vi "CSC-Remote_DisplayCSC.vi"(4 "AnkleTraj":dbl[][](array[numeric]), 5 "ClosePt":dbl[](array[numeric]), 6 "Init?":bool, 7 "Field Force":dbl[](array[numeric]), 8 "error in (no error)":errorcluster, 9 "AxisSetting":T1={"AxisLabel"=["x ", "y", "z "], "AxisMax"=[0.6, 0.7, 0.2], "AxisMin"=[-0.4, -0.3, -0.8]}, 10 "3D graph in":refnum<k7>, 11 "CSC in":refnum<class "CableSerialChain.lvclass">) -> (0 "error out":errorcluster, 1 "LastPlotNum":i32=1, 2 "3D graph out":refnum<k7>, 3 "CSC out":refnum<class "CableSerialChain.lvclass">)   [LabVIEW 2015, in "CSC-Remote.lvclass"]
uses:
  CSC-Remote.lvclass
  CableSerialChain/CableSerialChain.lvclass
  <vilib>/Platform/NI_3dgraph.lvlib
  <vilib>/ptbypt/NI_PtbyPt.lvlib
panel:
  out "EndEffInGCS":dbl[](array[numeric]) format="%#.6f"
  in  "sample length":i32=15
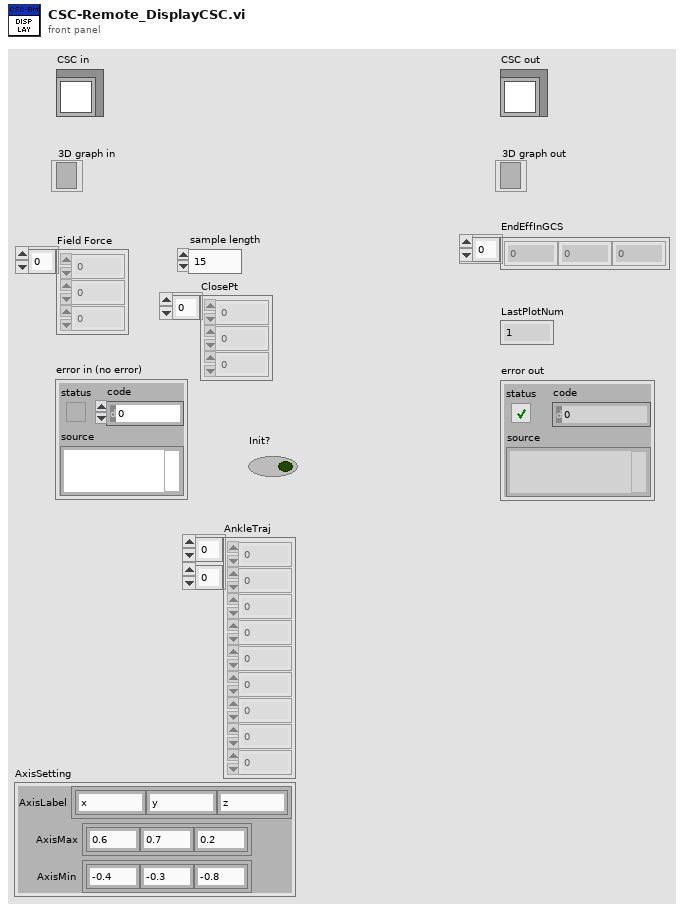
[diagram p1: front panel]
types:
  T1 = cluster{"AxisLabel":string[], "AxisMax":dbl[], "AxisMin":dbl[]}
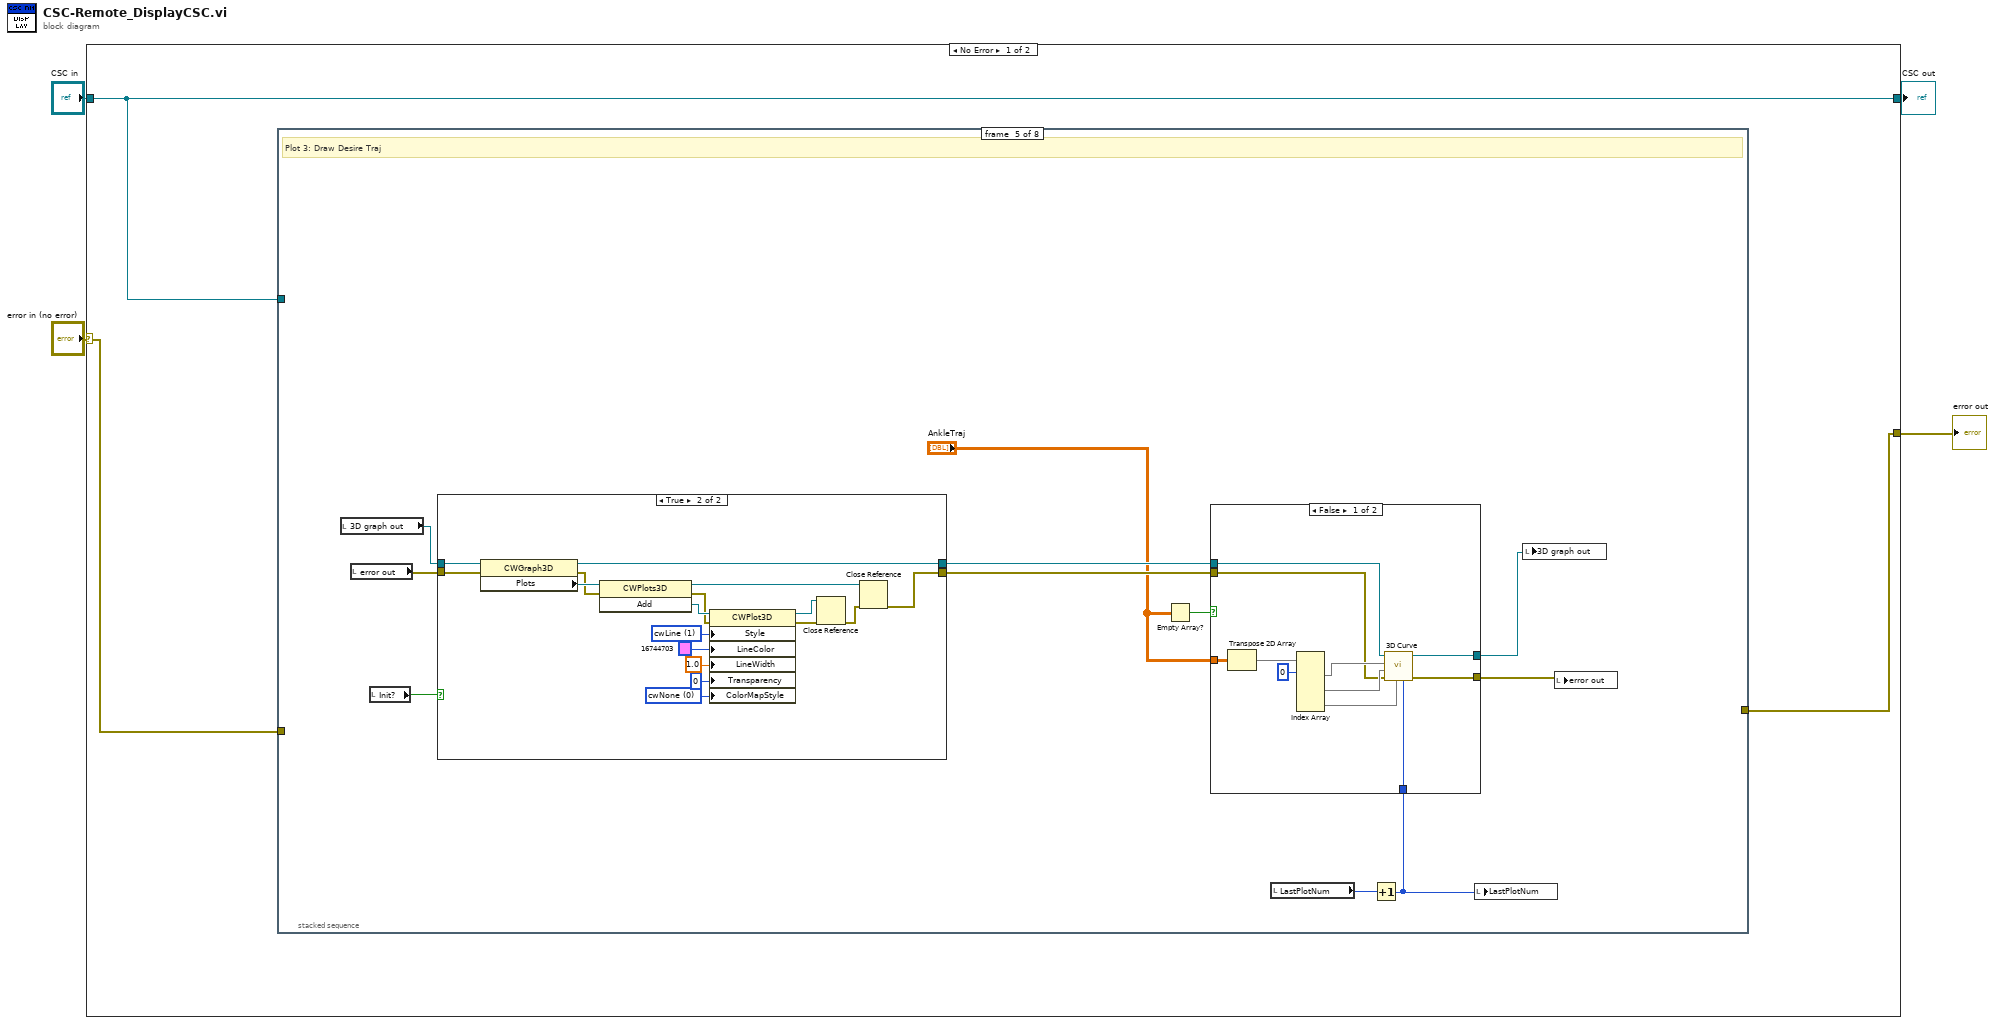
[diagram p0: block diagram]
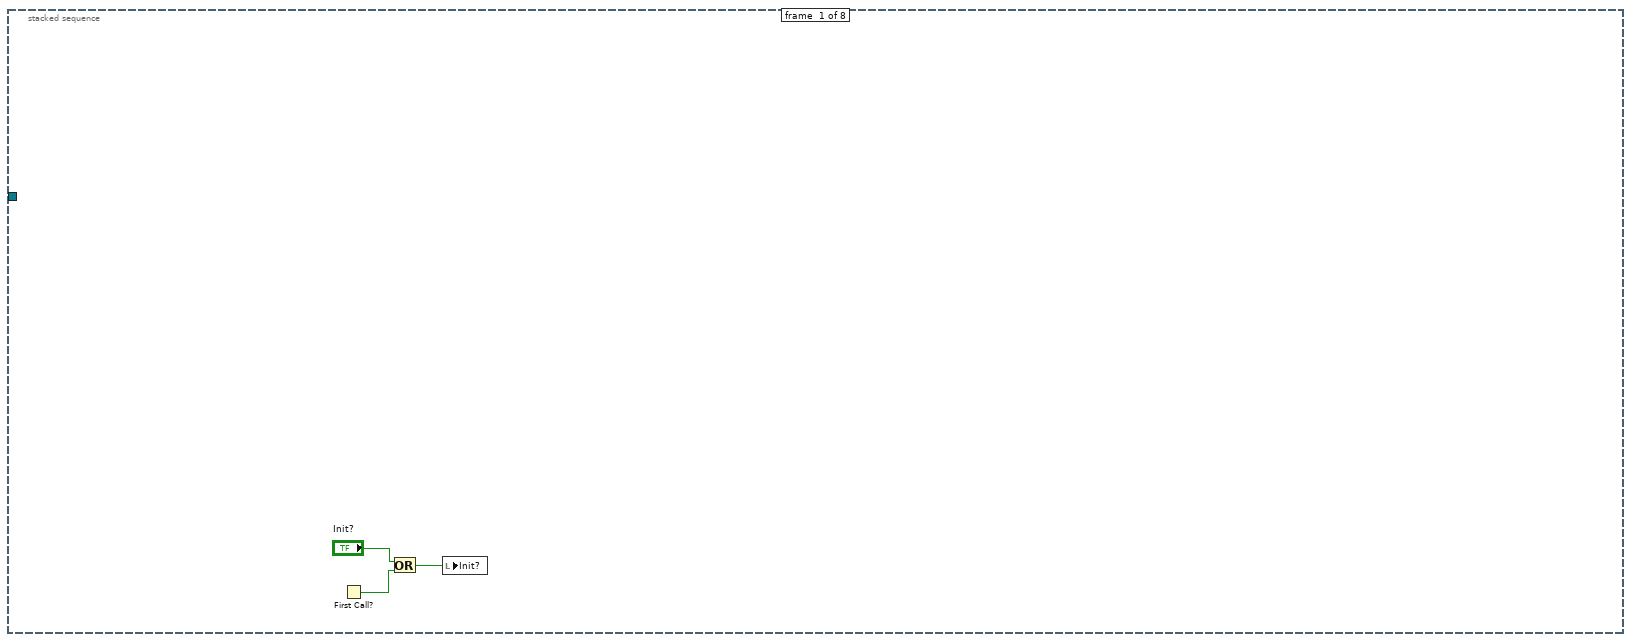
[diagram p2: hidden frame]
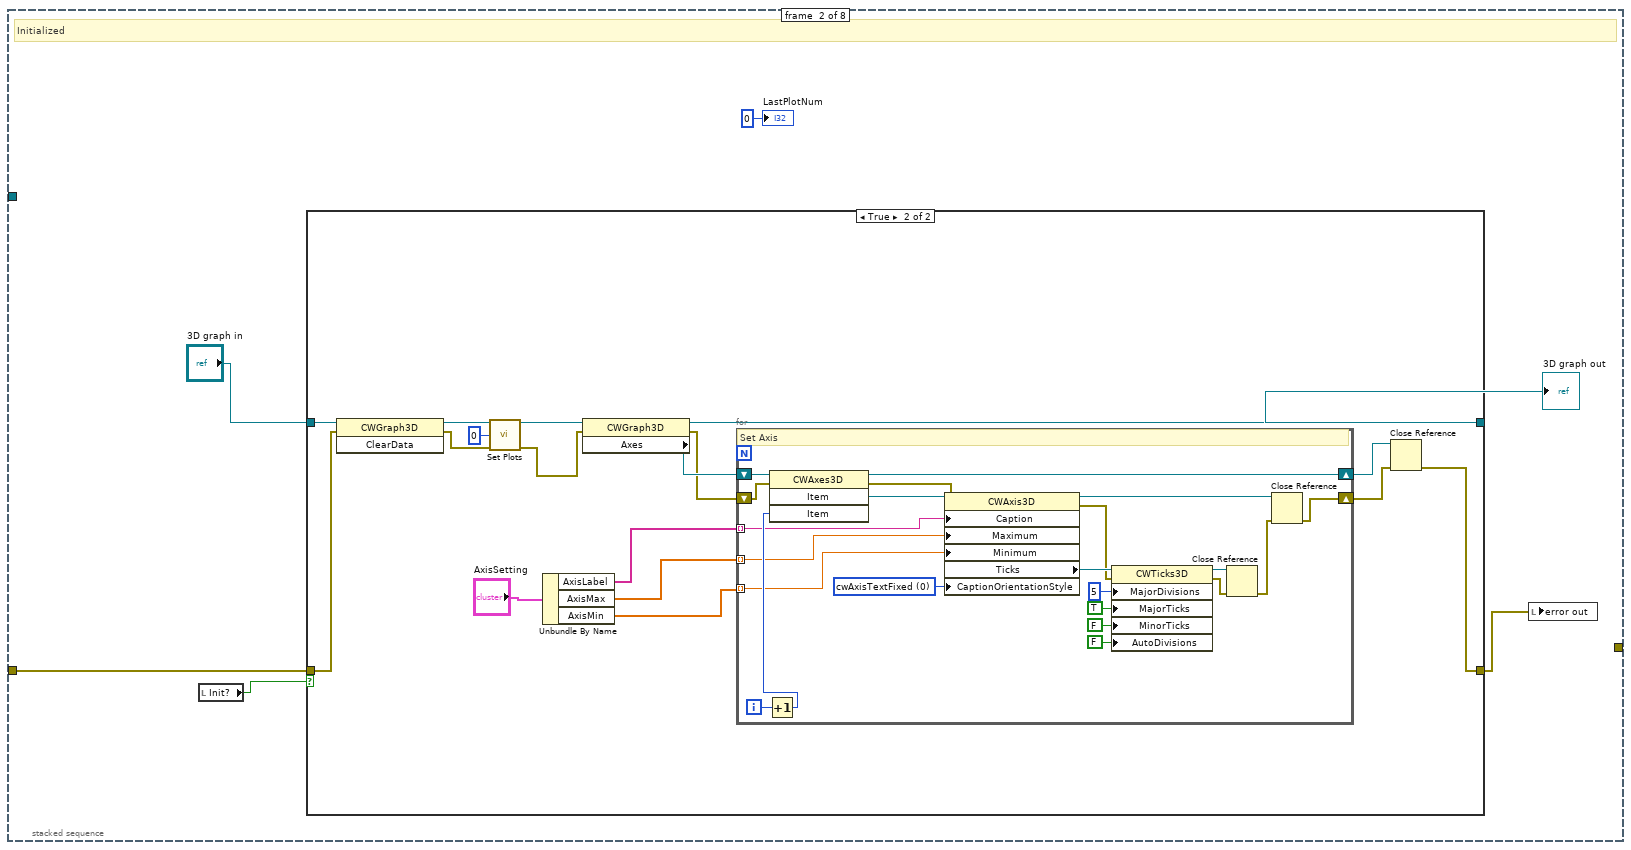
[diagram p3: hidden frame]
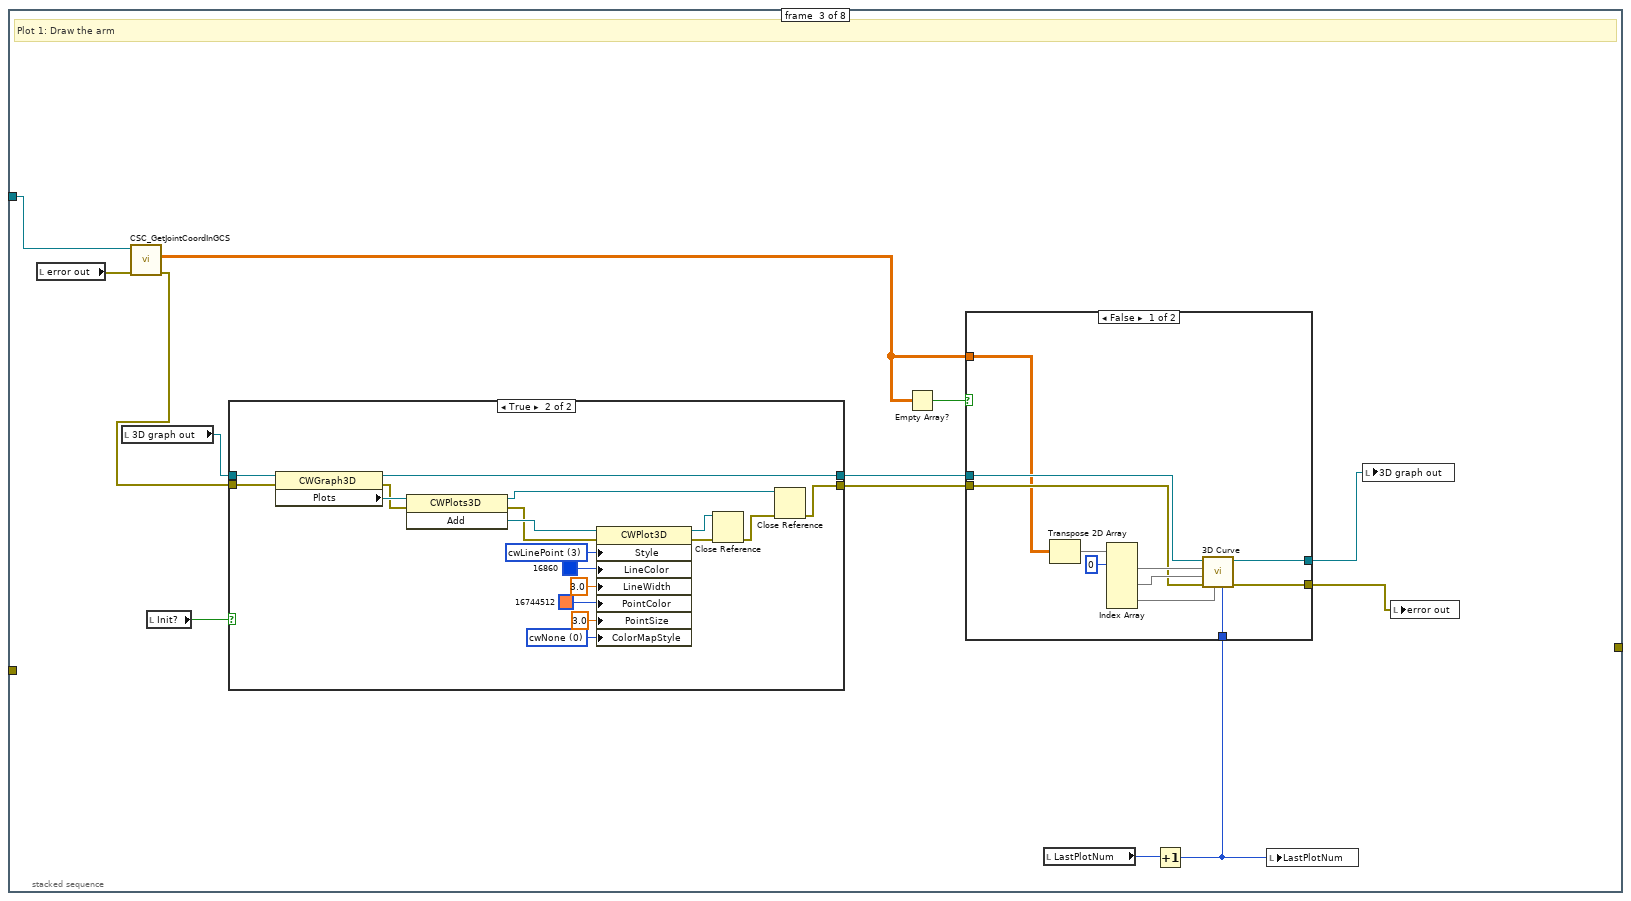
[diagram p5: hidden frame]
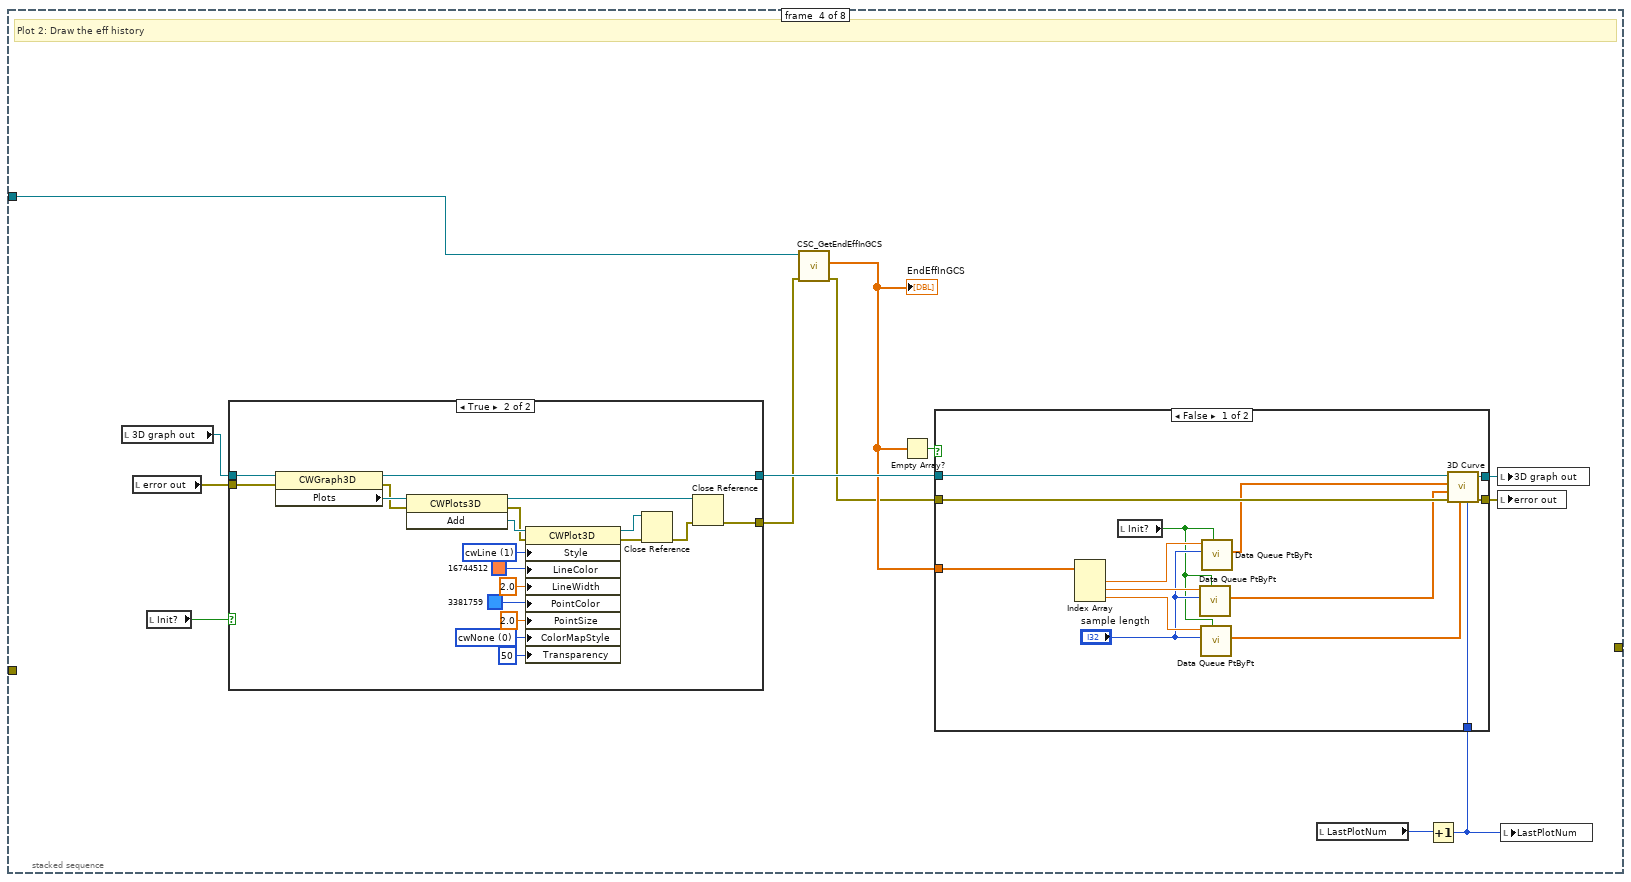
[diagram p8: hidden frame]
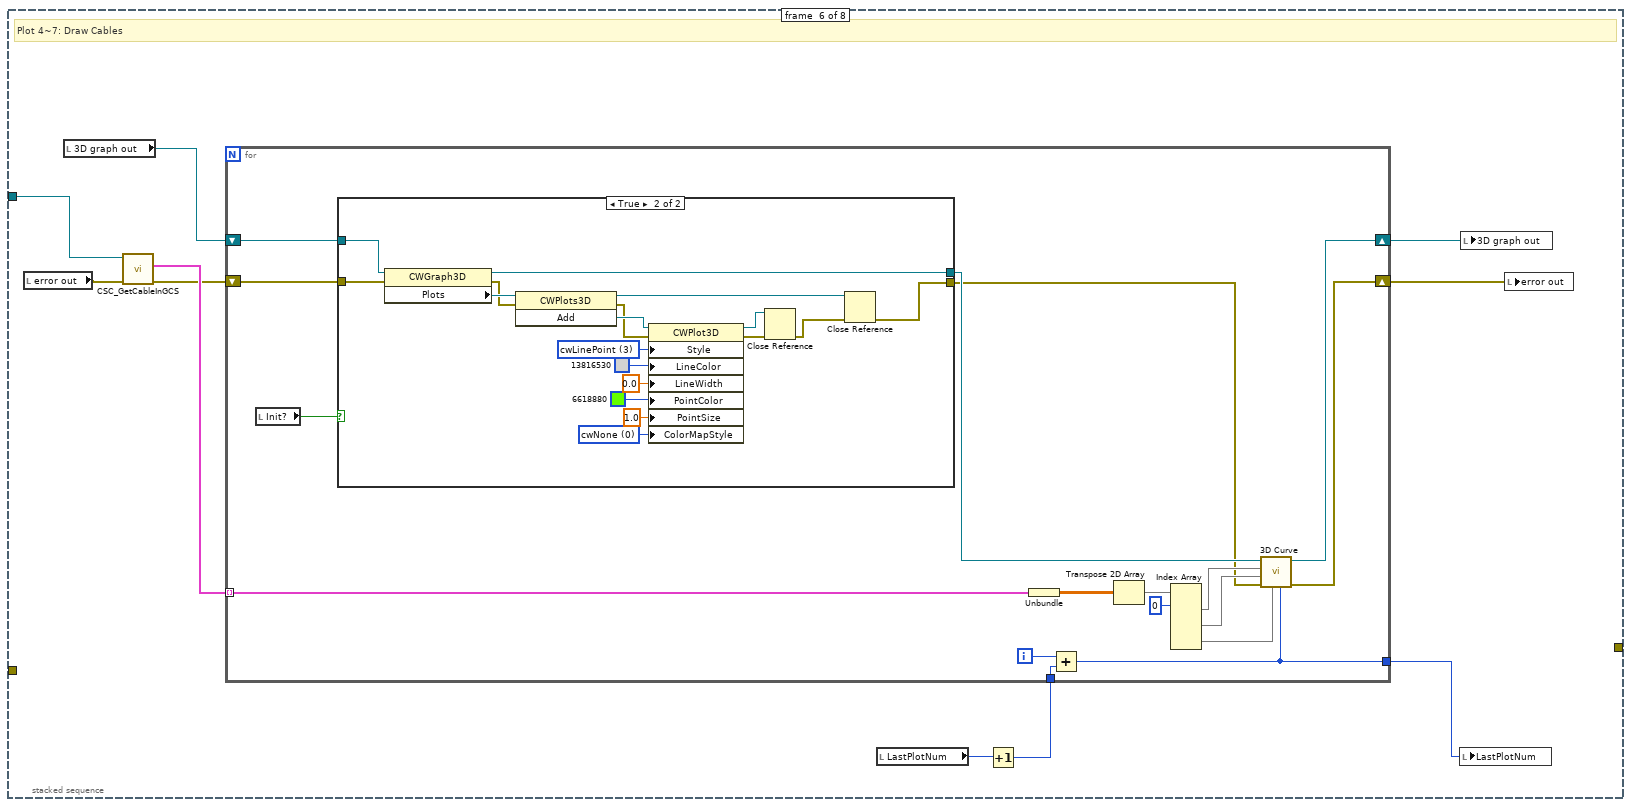
[diagram p13: hidden frame]
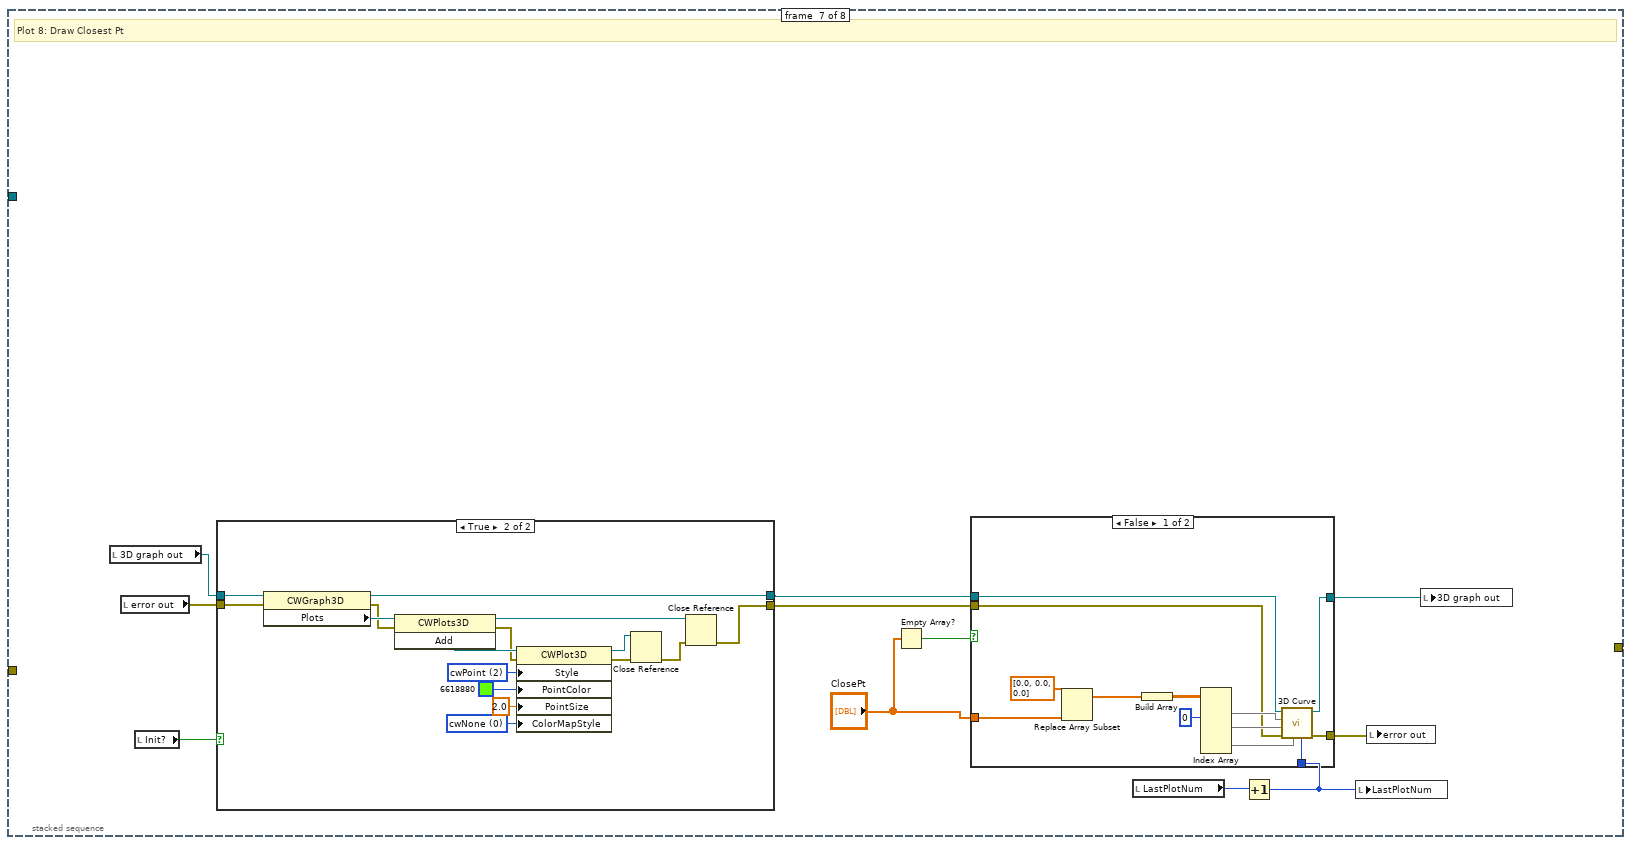
[diagram p15: hidden frame]
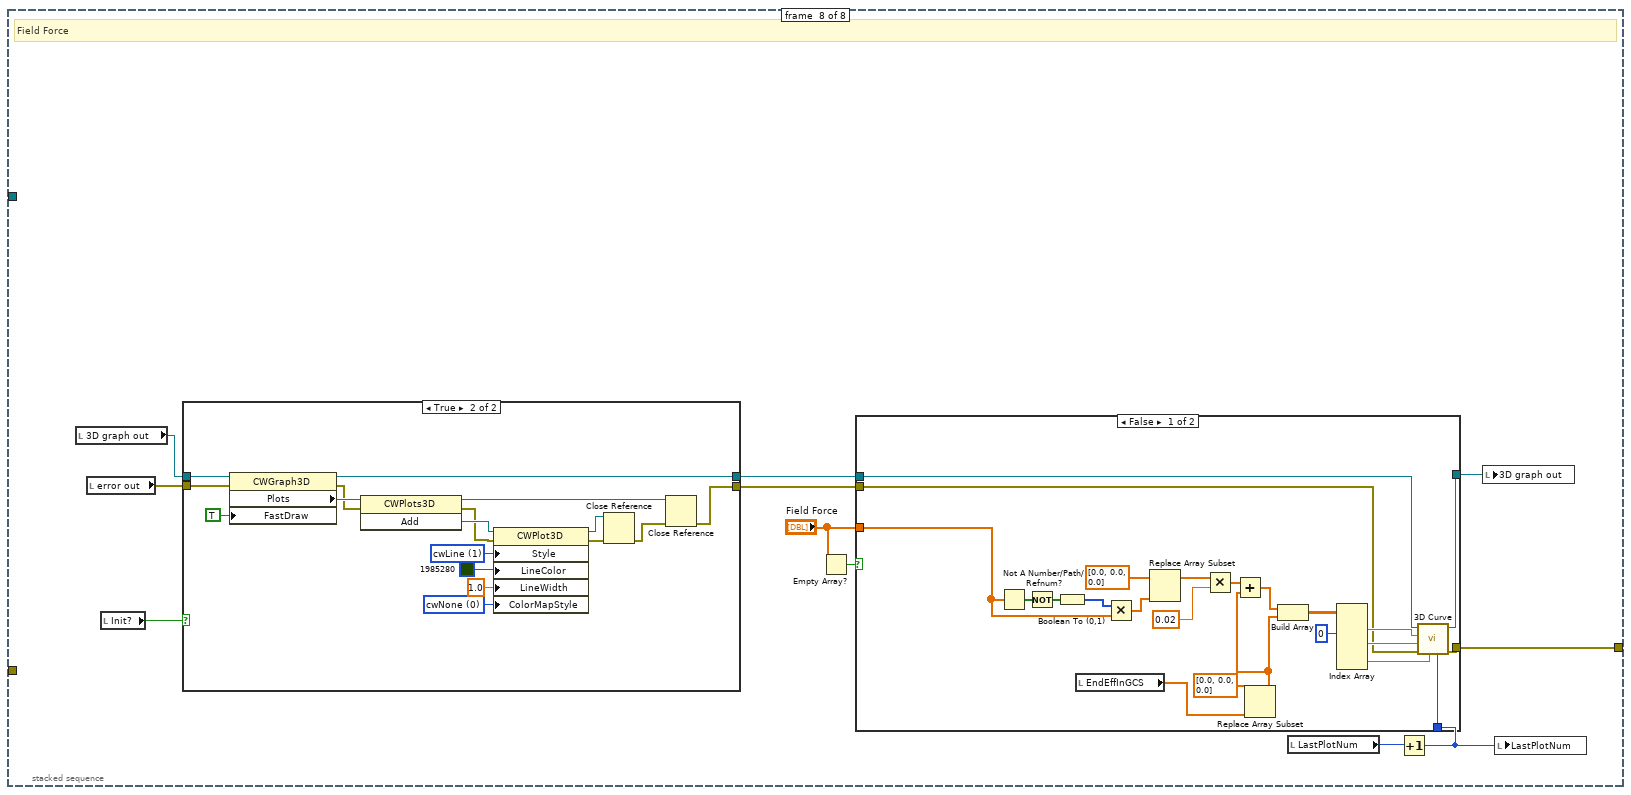
[diagram p18: hidden frame]
diagram:
  n1 = case shown="No Error" "error in (no error)" {
    selector: "error in (no error)" -> [w6 w344]
    tunnel: [w7 w344] -> w1
    tunnel: [w5 w343] -> w2
    tunnel: "CSC in" -> [w5 w343]
    frame No Error {
      n2 = stacked-sequence {
        tunnel: [_ _ _ _ _ _ _ w288] -> w7
        tunnel: w6 -> [_ w12 _ _ _ _ _ _]
        tunnel: w5 -> [_ _ w68 w116 _ w203 _ _]
        frame #0 {
          n3 = First Call?() -> (First Call?: T/F=w10:bool)
          n4 = Or(x="Init?", y=w10) -> (x .or. y?=w8:bool)
          n5 = local write "Init?"(w8) -> ()
        }
        frame #1 {
          # "Initialized"
          n6 = local read "Init?"() -> (w11:bool)
          n7 = case shown="True" w11 {
            tunnel: "3D graph in" -> [w18 w32]
            tunnel: [w18 w28] -> w15
            tunnel: [w17 w23] -> w13
            tunnel: w12 -> [w17 w30]
            frame False {
            }
            frame True {
              n8 = invoke class="CWGraph3D" method="ClearData"(reference=w32, error in=w30) -> (reference out=w31:refnum<k7>, error out=w29:errorcluster)  [unwired: 1 in, 1 out]
              n9 = call <vilib>:"Set Plots.vi"("3D graph"=w31, "# of plots(1)"=0, "error in (no error)"=w29) -> ("3D graph out"=w33:refnum<k7>, "error out"=w24:errorcluster)  [unwired: 11 in]
              n10 = Unbundle By Name("AxisSetting") -> ("AxisLabel"=w21:string[], "AxisMax"=w20:dbl[], "AxisMin"=w19:dbl[])
              n11 = property class="CWGraph3D"(reference=w33, error in=w24) -> (reference out=w28:refnum<k7>, error out=w25:errorcluster, "Axes"=w34:refnum<k7>)
              n12 = for {
                shift-right: [w44] -> w26
                shift-left: w34 -> [w57]
                shift-right: [w45] -> w27
                shift-left: w25 -> [w42]
                tunnel: w21 -> [w38] mode=indexing
                tunnel: w20 -> [w37] mode=indexing
                tunnel: w19 -> [w36] mode=indexing
                i -> [w40]
                w41 = 0 items=["cwAxisTextFixed", "cwAxisTextFaceCamera"] ("CaptionOrientationStyle")
                # "Set Axis"
                n13 = Increment(x=w40) -> (x+1=w39:i32)
                n14 = invoke class="CWAxes3D" method="Item"(reference=w57, error in=w42, "Item"=w39) -> (reference out=w44:refnum<k7>, error out=w43:errorcluster, "Item"=w56:refnum<k7>)  [unwired: 1 in, 1 out]
                n15 = property class="CWAxis3D"(reference=w56, error in=w43, "Caption"=w38, "Maximum"=w37, "Minimum"=w36, "CaptionOrientationStyle"=w41) -> (reference out=w46:refnum<k7>, error out=w49:errorcluster, "Ticks"=w55:refnum<k7>)
                n16 = property class="CWTicks3D"(reference=w55, error in=w49, "MajorDivisions"=5, "MajorTicks"=TRUE, "MinorTicks"=FALSE, "AutoDivisions"=FALSE) -> (reference out=w48:refnum<k7>, error out=w50:errorcluster)
                n17 = Close Reference(reference=w48, error in (no error)=w50) -> (error out=w47:errorcluster)
                n18 = Close Reference(reference=w46, error in (no error)=w47) -> (error out=w45:errorcluster)
              }
              n19 = Close Reference(reference=w26, error in (no error)=w27) -> (error out=w23:errorcluster)
            }
          }
          "3D graph out" <- w15
          n20 = local write "error out"(w13) -> ()
          "LastPlotNum" <- 0 ("LastPlotNum 2")
        }
        frame #2 {
          # "Plot 1: Draw the arm"
          n21 = local read "error out"() -> (w60:errorcluster)
          n22 = local read "3D graph out"() -> (w66:refnum<k7>)
          n23 = call "CSC_GetJointCoordInGCS.vi"("error in (no error)"=w60, "C-Alex in"=w68) -> ("error out"=w59:errorcluster, "Joint Coord in GCS"=w58:dbl[][])  [unwired: 6 in, 2 out]
          n24 = local read "Init?"() -> (w62:bool)
          n25 = case shown="True" w62 {
            tunnel: w59 -> [w84 w97]
            tunnel: w66 -> [w85 w92]
            tunnel: [w85 w91] -> w65
            tunnel: [w84 w86] -> w64
            frame False {
            }
            frame True {
              w90 = 0 items=["cwNone", "cwShaded", "cwColorSpectrum", "cwGrayScale", "cwCustom"] ("ColorMapStyle")
              w103 = 3 items=["cwLine"=1, "cwPoint"=2, "cwLinePoint"=3, "cwHiddenLine"=4, "cwSurface"=5, "cwSurfaceLine"=6, "cwSurfaceNormal"=7, "cwContourLine"=8, "cwSurfaceContour"=9] ("Style")
              n26 = property class="CWGraph3D"(reference=w92, error in=w97) -> (reference out=w91:refnum<k7>, error out=w100:errorcluster, "Plots"=w101:refnum<k7>)
              n27 = invoke class="CWPlots3D" method="Add"(reference=w101, error in=w100) -> (reference out=w88:refnum<k7>, error out=w89:errorcluster, "Add"=w102:refnum<k7>)  [unwired: 1 in]
              n28 = property class="CWPlot3D"(reference=w102, error in=w89, "Style"=w103, "LineColor"=u32 16860, "LineWidth"=3.0, "PointColor"=u32 16744512, "PointSize"=3.0 ("LineWidth"), "ColorMapStyle"=w90) -> (reference out=w98:refnum<k7>, error out=w99:errorcluster)
              n29 = Close Reference(reference=w98, error in (no error)=w99) -> (error out=w87:errorcluster)
              n30 = Close Reference(reference=w88, error in (no error)=w87) -> (error out=w86:errorcluster)
            }
          }
          n31 = Empty Array?(array=w58) -> (empty?=w61:bool)
          n32 = local read "LastPlotNum"() -> (w70:i32)
          n33 = Increment(x=w70) -> (x+1=w69:i32)
          n34 = case shown="False" w61 {
            tunnel: [w76 w83] -> w67
            tunnel: w65 -> [w75 w83]
            tunnel: w64 -> [w74 w82]
            tunnel: [w73 w82] -> w63
            tunnel: w69 -> [w72 _]
            tunnel: w58 -> [w71 _]
            frame False {
              n35 = Transpose 2D Array(2D array=w71) -> (transposed array=w77:dbl[][])
              n36 = Index Array(array=w77, index (row) #1=0 ("index (row)")) -> (element #1=w79:dbl[], element #2=w80:dbl[], element #3=w81:dbl[])  [unwired: 5 in]
              n37 = call <vilib>:"3D Curve.vi"("plot number (1)"=w72, "z vector"=w81, "error in (no error)"=w74, "y vector"=w80, "x vector"=w79, "3D graph"=w75) -> ("error out"=w73:errorcluster, "3D graph out"=w76:refnum<k7>)  [unwired: 4 in]
            }
            frame True {
            }
          }
          n38 = local write "LastPlotNum"(w69) -> ()
          n39 = local write "3D graph out"(w67) -> ()
          n40 = local write "error out"(w63) -> ()
        }
        frame #3 {
          # "Plot 2: Draw the eff history"
          n41 = local read "3D graph out"() -> (w111:refnum<k7>)
          n42 = local read "error out"() -> (w112:errorcluster)
          n43 = local read "Init?"() -> (w108:bool)
          n44 = case shown="True" w108 {
            tunnel: w112 -> [w133 w146]
            tunnel: w111 -> [w134 w141]
            tunnel: [w134 w140] -> w110
            tunnel: [w133 w135] -> w105
            frame False {
            }
            frame True {
              w139 = 0 items=["cwNone", "cwShaded", "cwColorSpectrum", "cwGrayScale", "cwCustom"] ("ColorMapStyle")
              w153 = 1 items=["cwLine"=1, "cwPoint"=2, "cwLinePoint"=3, "cwHiddenLine"=4, "cwSurface"=5, "cwSurfaceLine"=6, "cwSurfaceNormal"=7, "cwContourLine"=8, "cwSurfaceContour"=9] ("Style")
              n45 = property class="CWGraph3D"(reference=w141, error in=w146) -> (reference out=w140:refnum<k7>, error out=w150:errorcluster, "Plots"=w151:refnum<k7>)
              n46 = invoke class="CWPlots3D" method="Add"(reference=w151, error in=w150) -> (reference out=w149:refnum<k7>, error out=w137:errorcluster, "Add"=w152:refnum<k7>)  [unwired: 1 in]
              n47 = property class="CWPlot3D"(reference=w152, error in=w137, "Style"=w153, "LineColor"=u32 16744512, "LineWidth"=2.0, "PointColor"=u32 3381759, "PointSize"=2.0 ("LineWidth"), "ColorMapStyle"=w139, "Transparency"=50) -> (reference out=w147:refnum<k7>, error out=w148:errorcluster)
              n48 = Close Reference(reference=w147, error in (no error)=w148) -> (error out=w136:errorcluster)
              n49 = Close Reference(reference=w149, error in (no error)=w136) -> (error out=w135:errorcluster)
            }
          }
          n50 = call "CSC_GetEndEffInGCS.vi"("error in (no error)"=w105, "CSC in"=w116) -> ("error out"=w104:errorcluster, "EndEffInGCS"=w106:dbl[])  [unwired: 5 in, 3 out]
          "EndEffInGCS" <- w106
          n51 = Empty Array?(array=w106) -> (empty?=w107:bool)
          n52 = local read "LastPlotNum"() -> (w114:i32)
          n53 = Increment(x=w114) -> (x+1=w115:i32)
          n54 = case shown="False" w107 {
            tunnel: [w130 w132] -> w113
            tunnel: w110 -> [w129 w132]
            tunnel: w104 -> [w128 w131]
            tunnel: [w127 w131] -> w109
            tunnel: w115 -> [w126 _]
            tunnel: w106 -> [w117 _]
            frame False {
              n55 = Index Array(array=w117) -> (element #1=w123:dbl, element #2=w124:dbl, element #3=w125:dbl)  [unwired: 3 in]
              n56 = local read "Init?"() -> (w118:bool)
              n57 = call <vilib>:"Data Queue PtByPt.vi"("initialize"=w118, "sample length"="sample length", "input data point"=w124) -> ("Current Queue"=w120:dbl[])  [unwired: 4 in, 4 out]
              n58 = call <vilib>:"Data Queue PtByPt.vi"("initialize"=w118, "sample length"="sample length", "input data point"=w125) -> ("Current Queue"=w119:dbl[])  [unwired: 4 in, 4 out]
              n59 = call <vilib>:"Data Queue PtByPt.vi"("initialize"=w118, "sample length"="sample length", "input data point"=w123) -> ("Current Queue"=w121:dbl[])  [unwired: 4 in, 4 out]
              n60 = call <vilib>:"3D Curve.vi"("plot number (1)"=w126, "z vector"=w119, "error in (no error)"=w128, "y vector"=w120, "x vector"=w121, "3D graph"=w129) -> ("error out"=w127:errorcluster, "3D graph out"=w130:refnum<k7>)  [unwired: 4 in]
            }
            frame True {
            }
          }
          n61 = local write "3D graph out"(w113) -> ()
          n62 = local write "error out"(w109) -> ()
          n63 = local write "LastPlotNum"(w115) -> ()
        }
        frame #4 {
          # "Plot 3: Draw Desire Traj"
          n64 = local read "3D graph out"() -> (w160:refnum<k7>)
          n65 = local read "error out"() -> (w161:errorcluster)
          n66 = local read "Init?"() -> (w158:bool)
          n67 = case shown="True" w158 {
            tunnel: w161 -> [w178 w189]
            tunnel: w160 -> [w179 w186]
            tunnel: [w179 w185] -> w159
            tunnel: [w178 w180] -> w157
            frame False {
            }
            frame True {
              w183 = 0 items=["cwNone", "cwShaded", "cwColorSpectrum", "cwGrayScale", "cwCustom"] ("ColorMapStyle")
              w196 = 1 items=["cwLine"=1, "cwPoint"=2, "cwLinePoint"=3, "cwHiddenLine"=4, "cwSurface"=5, "cwSurfaceLine"=6, "cwSurfaceNormal"=7, "cwContourLine"=8, "cwSurfaceContour"=9] ("Style")
              n68 = property class="CWGraph3D"(reference=w186, error in=w189) -> (reference out=w185:refnum<k7>, error out=w193:errorcluster, "Plots"=w194:refnum<k7>)
              n69 = invoke class="CWPlots3D" method="Add"(reference=w194, error in=w193) -> (reference out=w192:refnum<k7>, error out=w182:errorcluster, "Add"=w195:refnum<k7>)  [unwired: 1 in]
              n70 = property class="CWPlot3D"(reference=w195, error in=w182, "Style"=w196, "LineColor"=u32 16744703, "LineWidth"=1.0, "Transparency"=0, "ColorMapStyle"=w183) -> (reference out=w190:refnum<k7>, error out=w191:errorcluster)
              n71 = Close Reference(reference=w190, error in (no error)=w191) -> (error out=w181:errorcluster)
              n72 = Close Reference(reference=w192, error in (no error)=w181) -> (error out=w180:errorcluster)
            }
          }
          n73 = Empty Array?(array="AnkleTraj") -> (empty?=w155:bool)
          n74 = local read "LastPlotNum"() -> (w164:i32)
          n75 = Increment(x=w164) -> (x+1=w163:i32)
          n76 = case shown="False" w155 {
            tunnel: "AnkleTraj" -> [w175 _]
            tunnel: [w169 w177] -> w162
            tunnel: w159 -> [w168 w177]
            tunnel: w163 -> [w167 _]
            tunnel: w157 -> [w166 w176]
            tunnel: [w165 w176] -> w156
            frame False {
              n77 = Transpose 2D Array(2D array=w175) -> (transposed array=w170:dbl[][])
              n78 = Index Array(array=w170, index (row) #1=0 ("index (row)")) -> (element #1=w172:dbl[], element #2=w173:dbl[], element #3=w174:dbl[])  [unwired: 5 in]
              n79 = call <vilib>:"3D Curve.vi"("plot number (1)"=w167, "z vector"=w174, "error in (no error)"=w166, "y vector"=w173, "x vector"=w172, "3D graph"=w168) -> ("error out"=w165:errorcluster, "3D graph out"=w169:refnum<k7>)  [unwired: 4 in]
            }
            frame True {
            }
          }
          n80 = local write "LastPlotNum"(w163) -> ()
          n81 = local write "3D graph out"(w162) -> ()
          n82 = local write "error out"(w156) -> ()
        }
        frame #5 {
          # "Plot 4~7: Draw Cables"
          n83 = local read "error out"() -> (w197:errorcluster)
          n84 = local read "3D graph out"() -> (w201:refnum<k7>)
          n85 = call "CSC_GetCableInGCS.vi"("error in (no error)"=w197, "C-Alex in"=w203) -> ("error out"=w198:errorcluster, "Cables Points"=w200:cluster{"PointInGCS":dbl[][]}[])  [unwired: 7 in, 1 out]
          n86 = local read "LastPlotNum"() -> (w206:i32)
          n87 = Increment(x=w206) -> (x+1=w205:i32)
          n88 = for {
            tunnel: w200 -> [w221] mode=indexing
            shift-right: [w219] -> w202
            shift-left: w201 -> [w213]
            tunnel: w205 -> [w211]
            tunnel: [w210] -> w204
            shift-right: [w208] -> w199
            shift-left: w198 -> [w207]
            i -> [w215]
            n89 = local read "Init?"() -> (w214:bool)
            n90 = case shown="True" w214 {
              tunnel: w207 -> [w225 w236]
              tunnel: [w224 w231] -> w212
              tunnel: [w225 w226] -> w209
              tunnel: w213 -> [w224 w229]
              frame False {
              }
              frame True {
                w230 = 0 items=["cwNone", "cwShaded", "cwColorSpectrum", "cwGrayScale", "cwCustom"] ("ColorMapStyle")
                w243 = 3 items=["cwLine"=1, "cwPoint"=2, "cwLinePoint"=3, "cwHiddenLine"=4, "cwSurface"=5, "cwSurfaceLine"=6, "cwSurfaceNormal"=7, "cwContourLine"=8, "cwSurfaceContour"=9] ("Style")
                n91 = property class="CWGraph3D"(reference=w229, error in=w236) -> (reference out=w231:refnum<k7>, error out=w240:errorcluster, "Plots"=w241:refnum<k7>)
                n92 = invoke class="CWPlots3D" method="Add"(reference=w241, error in=w240) -> (reference out=w239:refnum<k7>, error out=w228:errorcluster, "Add"=w242:refnum<k7>)  [unwired: 1 in]
                n93 = property class="CWPlot3D"(reference=w242, error in=w228, "Style"=w243, "LineColor"=u32 13816530, "LineWidth"=0.0, "PointColor"=u32 6618880, "PointSize"=1.0 ("LineWidth"), "ColorMapStyle"=w230) -> (reference out=w237:refnum<k7>, error out=w238:errorcluster)
                n94 = Close Reference(reference=w237, error in (no error)=w238) -> (error out=w227:errorcluster)
                n95 = Close Reference(reference=w239, error in (no error)=w227) -> (error out=w226:errorcluster)
              }
            }
            n96 = Unbundle(w221) -> ("PointInGCS"=w220:dbl[][])
            n97 = Add(x=w215, y=w211) -> (x+y=w210:i32)
            n98 = Transpose 2D Array(2D array=w220) -> (transposed array=w222:dbl[][])
            n99 = Index Array(array=w222, index (row) #1=0 ("index (row)")) -> (element #1=w218:dbl[], element #2=w217:dbl[], element #3=w216:dbl[])  [unwired: 5 in]
            n100 = call <vilib>:"3D Curve.vi"("plot number (1)"=w210, "z vector"=w216, "error in (no error)"=w209, "y vector"=w217, "x vector"=w218, "3D graph"=w212) -> ("error out"=w208:errorcluster, "3D graph out"=w219:refnum<k7>)  [unwired: 4 in]
          }
          n101 = local write "LastPlotNum"(w204) -> ()
          n102 = local write "3D graph out"(w202) -> ()
          n103 = local write "error out"(w199) -> ()
        }
        frame #6 {
          # "Plot 8: Draw Closest Pt"
          n104 = local read "3D graph out"() -> (w252:refnum<k7>)
          n105 = local read "error out"() -> (w253:errorcluster)
          n106 = local read "Init?"() -> (w251:bool)
          n107 = case shown="True" w251 {
            tunnel: w253 -> [w270 w280]
            tunnel: w252 -> [w271 w277]
            tunnel: [w271 w276] -> w250
            tunnel: [w270 w272] -> w247
            frame False {
            }
            frame True {
              w275 = 0 items=["cwNone", "cwShaded", "cwColorSpectrum", "cwGrayScale", "cwCustom"] ("ColorMapStyle")
              w287 = 2 items=["cwLine"=1, "cwPoint"=2, "cwLinePoint"=3, "cwHiddenLine"=4, "cwSurface"=5, "cwSurfaceLine"=6, "cwSurfaceNormal"=7, "cwContourLine"=8, "cwSurfaceContour"=9] ("Style")
              n108 = property class="CWGraph3D"(reference=w277, error in=w280) -> (reference out=w276:refnum<k7>, error out=w284:errorcluster, "Plots"=w285:refnum<k7>)
              n109 = invoke class="CWPlots3D" method="Add"(reference=w285, error in=w284) -> (reference out=w283:refnum<k7>, error out=w274:errorcluster, "Add"=w286:refnum<k7>)  [unwired: 1 in]
              n110 = property class="CWPlot3D"(reference=w286, error in=w274, "Style"=w287, "PointColor"=u32 6618880, "PointSize"=2.0 ("LineWidth"), "ColorMapStyle"=w275) -> (reference out=w281:refnum<k7>, error out=w282:errorcluster)
              n111 = Close Reference(reference=w281, error in (no error)=w282) -> (error out=w273:errorcluster)
              n112 = Close Reference(reference=w283, error in (no error)=w273) -> (error out=w272:errorcluster)
            }
          }
          n113 = Empty Array?(array="ClosePt") -> (empty?=w244:bool)
          n114 = local read "LastPlotNum"() -> (w249:i32)
          n115 = Increment(x=w249) -> (x+1=w248:i32)
          n116 = case shown="False" w244 {
            tunnel: "ClosePt" -> [w266 _]
            tunnel: [w259 w269] -> w254
            tunnel: w250 -> [w258 w269]
            tunnel: w248 -> [w257 _]
            tunnel: w247 -> [w256 w268]
            tunnel: [w255 w268] -> w246
            frame False {
              n117 = Replace Array Subset(array=dbl[] [0.0, 0.0, 0.0], new element=w266) -> (w265:dbl[])  [unwired: 1 in]
              n118 = Build Array(w265) -> (w264:dbl[][])
              n119 = Index Array(array=w264, index (col) #1=0 ("disabled index (col)")) -> (element #1=w262:dbl[], element #2=w261:dbl[], element #3=w260:dbl[])  [unwired: 5 in]
              n120 = call <vilib>:"3D Curve.vi"("plot number (1)"=w257, "z vector"=w260, "error in (no error)"=w256, "y vector"=w261, "x vector"=w262, "3D graph"=w258) -> ("error out"=w255:errorcluster, "3D graph out"=w259:refnum<k7>)  [unwired: 4 in]
            }
            frame True {
            }
          }
          n121 = local write "LastPlotNum"(w248) -> ()
          n122 = local write "error out"(w246) -> ()
          n123 = local write "3D graph out"(w254) -> ()
        }
        frame #7 {
          # "Field Force"
          n124 = local read "3D graph out"() -> (w296:refnum<k7>)
          n125 = local read "error out"() -> (w297:errorcluster)
          n126 = local read "Init?"() -> (w295:bool)
          n127 = case shown="True" w295 {
            tunnel: w297 -> [w324 w335]
            tunnel: w296 -> [w325 w332]
            tunnel: [w325 w331] -> w294
            tunnel: [w324 w326] -> w291
            frame False {
            }
            frame True {
              w330 = 0 items=["cwNone", "cwShaded", "cwColorSpectrum", "cwGrayScale", "cwCustom"] ("ColorMapStyle")
              w342 = 1 items=["cwLine"=1, "cwPoint"=2, "cwLinePoint"=3, "cwHiddenLine"=4, "cwSurface"=5, "cwSurfaceLine"=6, "cwSurfaceNormal"=7, "cwContourLine"=8, "cwSurfaceContour"=9] ("Style")
              n128 = property class="CWGraph3D"(reference=w332, error in=w335, "FastDraw"=TRUE) -> (reference out=w331:refnum<k7>, error out=w339:errorcluster, "Plots"=w340:refnum<k7>)
              n129 = invoke class="CWPlots3D" method="Add"(reference=w340, error in=w339) -> (reference out=w338:refnum<k7>, error out=w328:errorcluster, "Add"=w341:refnum<k7>)  [unwired: 1 in]
              n130 = property class="CWPlot3D"(reference=w341, error in=w328, "Style"=w342, "LineColor"=u32 1985280, "LineWidth"=1.0, "ColorMapStyle"=w330) -> (reference out=w336:refnum<k7>, error out=w337:errorcluster)
              n131 = Close Reference(reference=w336, error in (no error)=w337) -> (error out=w327:errorcluster)
              n132 = Close Reference(reference=w338, error in (no error)=w327) -> (error out=w326:errorcluster)
            }
          }
          n133 = Empty Array?(array="Field Force") -> (empty?=w289:bool)
          n134 = local read "LastPlotNum"() -> (w293:i32)
          n135 = Increment(x=w293) -> (x+1=w292:i32)
          n136 = case shown="False" w289 {
            tunnel: [w305 w323] -> w298
            tunnel: w294 -> [w304 w323]
            tunnel: w292 -> [w303 _]
            tunnel: w291 -> [w302 w322]
            tunnel: [w301 w322] -> w288
            tunnel: "Field Force" -> [w300 _]
            frame False {
              n137 = Not A Number/Path/Refnum?(number/path/refnum=w300) -> (NaN/Path/Refnum?=w309:bool[])
              n138 = Not(x=w309) -> (.not. x?=w308:bool[])
              n139 = Boolean To (0,1)(Boolean=w308) -> (0, 1=w307:i16[])
              n140 = local read "EndEffInGCS"() -> (w299:dbl[])
              n141 = Multiply(x=w307, y=w300) -> (x*y=w306:dbl[])
              n142 = Replace Array Subset(array=dbl[] [0.0, 0.0, 0.0], new element=w306) -> (w319:dbl[])  [unwired: 1 in]
              n143 = Multiply(x=w319, y=0.02) -> (x*y=w314:dbl[])
              n144 = Replace Array Subset(array=dbl[] [0.0, 0.0, 0.0], new element=w299) -> (w321:dbl[])  [unwired: 1 in]
              n145 = Add(x=w314, y=w321) -> (x+y=w311:dbl[])
              n146 = Build Array(w311, w321) -> (w312:dbl[][])
              n147 = Index Array(array=w312, index (col) #1=0 ("disabled index (col)")) -> (element #1=w315:dbl[], element #2=w316:dbl[], element #3=w317:dbl[])  [unwired: 5 in]
              n148 = call <vilib>:"3D Curve.vi"("plot number (1)"=w303, "z vector"=w317, "error in (no error)"=w302, "y vector"=w316, "x vector"=w315, "3D graph"=w304) -> ("error out"=w301:errorcluster, "3D graph out"=w305:refnum<k7>)  [unwired: 4 in]
            }
            frame True {
            }
          }
          n149 = local write "3D graph out"(w298) -> ()
          n150 = local write "LastPlotNum"(w292) -> ()
        }
      }
    }
    frame Error {
    }
  }
  "CSC out" <- w2
  "error out" <- w1
